vi "Start Sequence Execution.vi"(8 "error in (no error)":errorcluster, 11 "teststand-api in":refnum<class "teststand-api.lvclass">) -> (0 "error out":errorcluster, 3 "teststand-api out":refnum<class "teststand-api.lvclass">)   [LabVIEW 2014, in "teststand-api.lvlib" / "teststand-api.lvclass"]
uses:
  teststand-api.lvclass
  teststand-api.lvclass/teststand-api.ctl
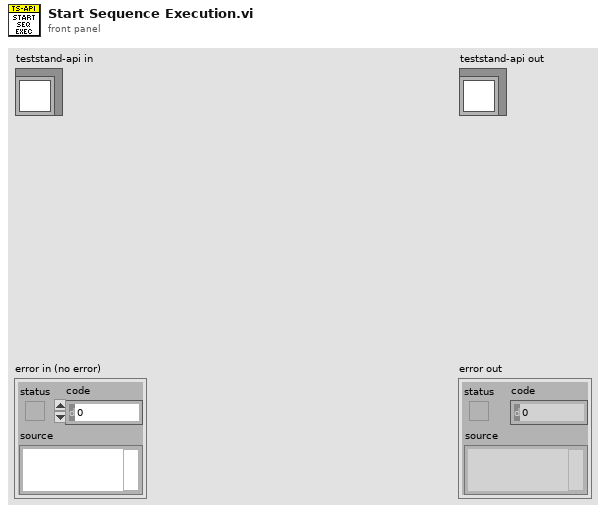
[diagram p1: front panel]
types:
  T1 = typedef "teststand-api.lvlib/teststand-api.lvclass/Model Run Mode--enum.ctl" = enum16{"Test UUTs", "Single Pass"}
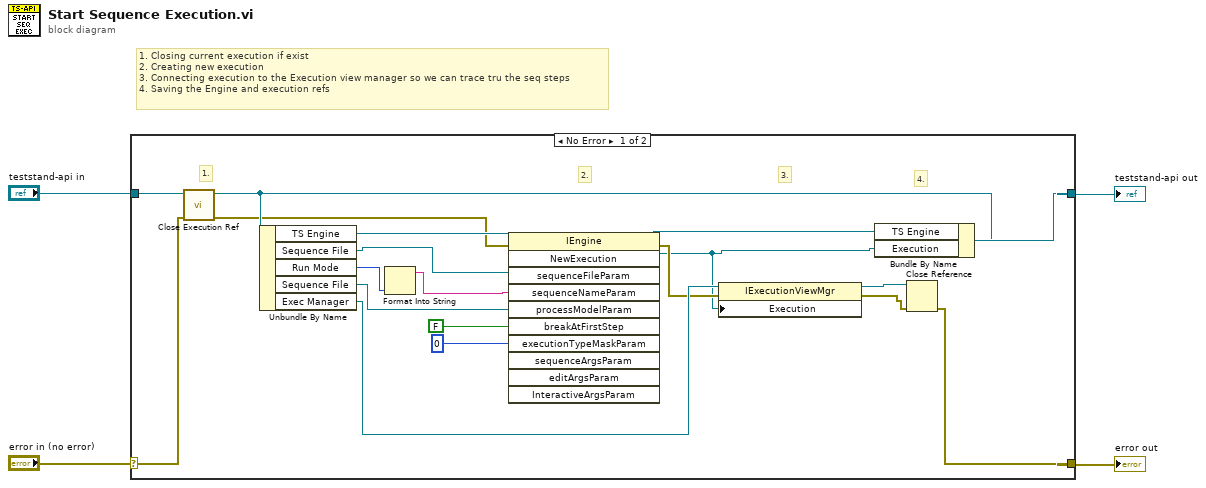
[diagram p0: block diagram]
diagram:
  # "1. Closing current execution if exist\n2. Creating new execution\n3. Connecting execution to the Execution view manager so we can trace tru the seq steps\n4. Saving the Engine and execution refs"
  n1 = case shown="No Error" "error in (no error)" {
    selector: "error in (no error)" -> [w6 w25]
    tunnel: [w9 w25] -> w3
    tunnel: [w22 w24] -> w1
    tunnel: "teststand-api in" -> [w8 w24]
    frame No Error {
      # "4."
      # "3."
      # "2."
      # "1."
      n2 = call-dynamic "Close Execution Ref.vi"("error in (no error)"=w6, "teststand-api in"=w8) -> ("error out"=w5:errorcluster, "teststand-api out"=w7:refnum<class "teststand-api.lvclass">)  [unwired: 8 in]
      n3 = Unbundle By Name(w7) -> ("TS Engine"=w23:refnum<k7>, "Sequence File"=w21:refnum<k7>, "Run Mode"=w20:T1, "Sequence File"=w18:refnum<k7>, "Exec Manager"=w14:refnum<k7>)
      n4 = Format Into String(w20) -> (resulting string=w19:string)  [unwired: 3 in, 1 out]
      n5 = invoke class="IEngine" method="NewExecution"(reference=w23, error in=w5, "sequenceFileParam"=w21, "sequenceNameParam"=w19, "processModelParam"=w18, "breakAtFirstStep"=FALSE, "executionTypeMaskParam"=0) -> (reference out=w15:refnum<k7>, error out=w13:errorcluster, "NewExecution"=w12:refnum<k7>)  [unwired: 4 in, 8 out]
      n6 = property class="IExecutionViewMgr"(reference=w14, error in=w13, "Execution"=w12) -> (reference out=w11:refnum<k7>, error out=w10:errorcluster)
      n7 = Bundle By Name(cluster=w7, "TS Engine"=w15, "Execution"=w12) -> (w22:refnum<class "teststand-api.lvclass">)
      n8 = Close Reference(reference=w11, error in (no error)=w10) -> (error out=w9:errorcluster)
    }
    frame Error {
    }
  }
  "error out" <- w3
  "teststand-api out" <- w1
